vi "Set Wheel Separation.vi"(8 "error in (no error)":errorcluster, 10 "wheel separation":dbl, 11 "differential steering frame in":refnum<class "NI_Robotics_Differential Steering Frame.lvclass">) -> (0 "error out":errorcluster, 3 "differential steering frame out":refnum<class "NI_Robotics_Differential Steering Frame.lvclass">)   [LabVIEW 2017, in "NI_Robotics_Differential Steering Frame.lvclass"]
uses:
  <vilib>/robotics/Steering/Differential Steering Frame/NI_Robotics_Differential Steering Frame.lvclass
  c:/Program Files (x86)/National Instruments/LabVIEW 2017/vi.lib/robotics/Steering/Steering Frame/NI_Robotics_Steering Frame.lvclass
  <vilib>/robotics/Steering/Steering Frame/NI_Robotics_Steering Frame.lvclass/NI_Robotics_Steering Frame.ctl
  <vilib>/robotics/Steering/Wheel/NI_Robotics_Wheel.lvclass/NI_Robotics_Wheel.ctl
  <vilib>/robotics/Steering/Differential Steering Frame/NI_Robotics_Differential Steering Frame.lvclass/NI_Robotics_Differential Steering Frame.ctl
  <vilib>/robotics/Steering/Wheel/Update Steering to Wheel Frame Transform.vi
  <vilib>/Analysis/coordinate.llb/Wrap Angle.vi
  <vilib>/Analysis/coordinate.llb/Wrap Angle (scalar).vi
  <vilib>/robotics/Steering/Steering Frame/NI_Robotics_Steering Frame.lvclass
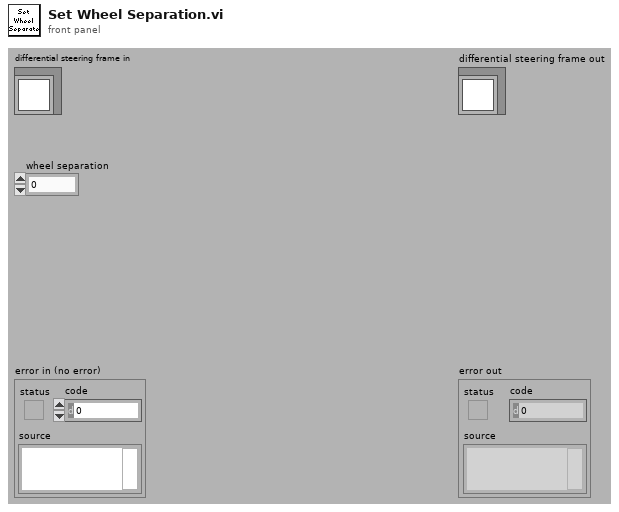
[diagram p1: front panel]
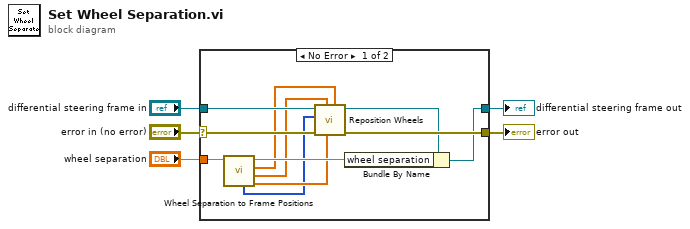
[diagram p0: block diagram]
diagram:
  n1 = case shown="No Error" "error in (no error)" {
    selector: "error in (no error)" -> [w15 w18]
    tunnel: [w14 w18] -> w4
    tunnel: [w12 w17] -> w2
    tunnel: "differential steering frame in" -> [w16 w17]
    tunnel: "wheel separation" -> [w11 _]
    frame No Error {
      n2 = call <vilib>:"Wheel Separation to Frame Positions.vi"("wheel separation"=w11) -> ("wheel frame angles (rad)"=w7:dbl[], "wheel y positions"=w8:dbl[], "wheel x positions"=w9:dbl[], "coerced wheel separation"=w10:dbl, "wheel indexes"=w6:i32[])  [unwired: 6 in]
      n3 = call <vilib>:"Reposition Wheels.vi"("x positions"=w9, "frame angles (rad)"=w7, "y positions"=w8, "error in (no error)"=w15, "wheel indexes"=w6, "steering frame in"=w16) -> ("error out"=w14:errorcluster, "steering frame out"=w13:refnum<class "NI_Robotics_Differential Steering Frame.lvclass">)  [unwired: 3 in, 1 out]
      n4 = Bundle By Name(cluster=w13, "wheel separation"=w10) -> (w12:refnum<class "NI_Robotics_Differential Steering Frame.lvclass">)
    }
    frame Error {
    }
  }
  "error out" <- w4
  "differential steering frame out" <- w2
